vi "msgDetailsToJSON.vi"(8 "error in (no error)":errorcluster, 9 "msgTypeEnum":T1, 10 "msgTypeDef":T2={"msgName"="move", "msgDetails"="\"tolerance\":2,"}, 11 "TcpServer.lvclass":refnum<class "TcpServer.lvclass">) -> (0 "error out":errorcluster, 2 "JSON string":string, 3 "TcpServer.lvclass":refnum<class "TcpServer.lvclass">)   [LabVIEW 2018, in "TcpServer.lvclass"]
doc: "Convert the msgName and msgDetails into JSON string, to be sent to TCP Client.\n\nNOTE: Do not call this directly.This is for internal use only."
uses:
  TcpServer.lvclass
  typedef/msgTypeDef.ctl
  typedef/msgTypeEnum.ctl
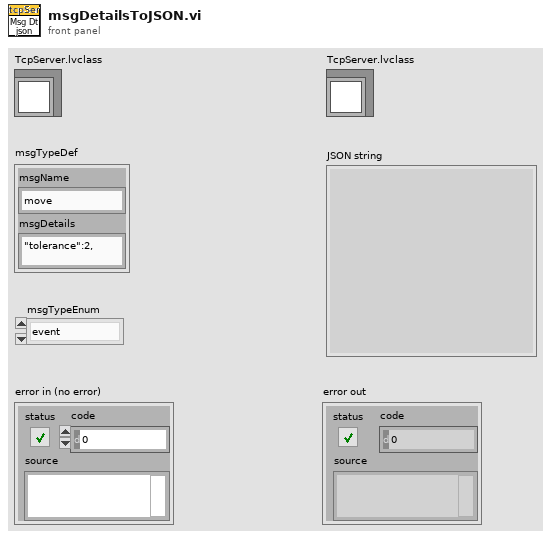
[diagram p1: front panel]
types:
  T1 = typedef "TcpServer.lvclass/msgTypeEnum.ctl" = enum16{"event", "telemetry"}
  T2 = typedef "TcpServer.lvclass/msgTypeDef.ctl" = cluster{"msgName":string, "msgDetails":string}
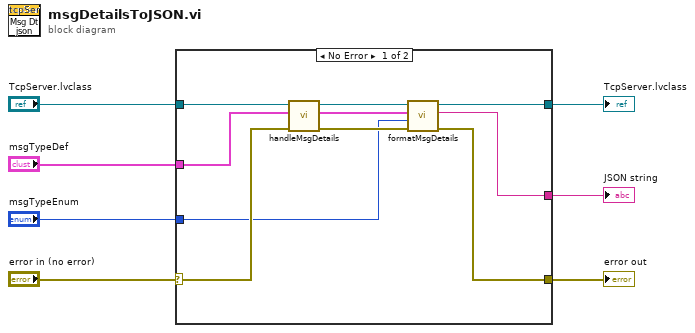
[diagram p0: block diagram]
diagram:
  n1 = case shown="No Error" "error in (no error)" {
    selector: "error in (no error)" -> [w12 w18]
    tunnel: "TcpServer.lvclass" -> [w16 w19]
    tunnel: [w14 w19] -> w6
    tunnel: [w13 _] -> w5
    tunnel: [w11 w18] -> w3
    tunnel: "msgTypeDef" -> [w9 _]
    tunnel: "msgTypeEnum" -> [w10 _]
    frame No Error {
      n2 = call "handleMsgDetails.vi"("error in (no error)"=w12, "msgTypeDef in"=w9, "TcpServer.lvclass"=w16) -> ("error out"=w17:errorcluster, "msgTypeDef out"=w8:T2, "TcpServer.lvclass"=w15:refnum<class "TcpServer.lvclass">)  [unwired: 6 in]
      n3 = call "formatMsgDetails.vi"("error in (no error)"=w17, "msgTypeEnum"=w10, "msgCluster"=w8, "TcpServer.lvclass"=w15) -> ("error out"=w11:errorcluster, "jsonString"=w13:string, "TcpServer.lvclass"=w14:refnum<class "TcpServer.lvclass">)  [unwired: 5 in]
    }
    frame Error {
    }
  }
  "JSON string" <- w5
  "TcpServer.lvclass" <- w6
  "error out" <- w3
